vi "Test Front Panel.vi"() -> ()   [LabVIEW 2018]
uses:
  Controls/Gauge TDef.ctl
  Controls/BlockStart Button.ctl
  Controls/BlockEnd Button.ctl
  Controls/GUI_Buttons_23x22_W2K.llb/MacroPlay.ctl
  Controls/GUI_Buttons_23x22_W2K.llb/MacroPause.ctl
  Controls/GUI_Buttons_23x22_W2K.llb/MacroStop.ctl
  Controls/GUI_Buttons_23x22_W2K.llb/Delete1.ctl
  Controls/GUI_Buttons_23x22_W2K.llb/EditGroup_1.ctl
  Controls/GUI_Buttons_23x22_W2K.llb/Cut.ctl
  Controls/GUI_Buttons_23x22_W2K.llb/Copy.ctl
  Controls/GUI_Buttons_23x22_W2K.llb/Paste.ctl
  Controls/GUI_Buttons_23x22_W2K.llb/FileGroup_1.ctl
  Controls/GUI_Buttons_23x22_W2K.llb/New.ctl
  Controls/GUI_Buttons_23x22_W2K.llb/Open.ctl
  Controls/GUI_Buttons_23x22_W2K.llb/Save.ctl
  Controls/Timing Mode.ctl
  Enable Controls API.llb/Action.ctl
  Enable Controls.lvlib
panel:
  out "PID Control Within Tolerance":bool
  out "Flow Meter":bool
  out "Thermocouple":bool
  out "Agilent":bool
  out "DAQ":bool
  in  "Rest All IO":bool
  in  "Exit":bool
  in  "Tab Control":T1(tab)
  in  "Go to Next Step":bool
  in  "BP Regulator Manual Control":bool
  in  "Current Manual Control":bool caption="Current Enabled"
  in  "Open Config":bool
  in  "Delete Config":bool
  in  "New Config":bool
  in  "Current Configration File":u16(ring) items=["Default"]
  out "Actual  Voltage":dbl(slide) scale=0.0..20.0 scale format="%#_g V"
  out "Current File Name":string
  out "Actual Current":dbl(slide) scale=0.0..360.0 scale format="%#_g mA"
  in  "Control Devices":cluster{"Current":dbl, "BP Regulator":dbl} {"BP Regulator" scale=0.0..300.0 scale format="%#3_0f psig"; "Current" scale=0.0..300.0 scale format="%#_g mA"}
  out "Test Status":T2(ring)
  out "Analog Sensors":T3 {"Fuel Temp" scale=0.0..150.0 scale format="%#.1f"; "Flow(lbs/hr)" scale=0.0..1000.0 scale format="%#.1f"; "BP Monitor" scale=0.0..10.0 scale format="%#.1f"; "Bypass Pressure (psig)" scale=0.0..50.0 scale format="%#.1f"; "(Not Used)" scale=0.0..200.0 scale format="%#.1f"; "Back Pressure" scale=0.0..300.0 scale format="%#.1f"; "Diff. Pressure  (60 psid)" scale=0.0..60.0 scale format="%#.1f"; "Supply Pressure" scale=0.0..400.0 scale format="%#.1f"}
  in  "BlkMrkGrp":cluster{"Block Start":T4, "Block End":T5}
  in  "MacroGroup":T9
  in  "Delete":T10
  in  "EditGroup_1":T11
  in  "FileGroup_1":T15
  in  "Test Table":string[][](table)=[["", "20", "10", "109 ", "200", " ", " ", " ", " ", " ", " ", " ", " ", " ", " "], ["", "40", "22", "160", "200", "", " ", " ", " ", " ", " ", " ", " ", " ", " "], ["", "10", "32", "400", "500", "", " ", " ", " ", " ", " ", " ", " ", " ", " "]] caption="Current         Dwell            Min Flow       Max Flow        Actual Flow    Hysteresis"
  out "EditLine":i32=65534
  out "EditCol":i32=65534
  in  "StartTest":bool
  in  "StopTest":bool
  in  "PauseTest":bool
  out "CountDown Pie":picture
  out "CountDown Text":string="0:00"
  in  "Test Timing Mode":T19
  in  "Send to Excel":bool
  in  "Additional Report Values":cluster{"Excel  Name":string, "Value":string}[](array[cluster])
  out "Test Table2":string[][](table)=[["", "20", "10", "109 ", "200", " ", " ", " ", " ", " ", " ", " ", " ", " ", " "], ["", "40", "22", "160", "200", "", " ", " ", " ", " ", " ", " ", " ", " ", " "], ["", "10", "32", "400", "500", "", " ", " ", " ", " ", " ", " ", " ", " ", " "]] caption="Table"
  in  "template (empty)":path
  out "Parameter Table Out":string[][](table)
  out "Flow-Current XY Graph":cluster{cluster{"X":dbl, "Y":dbl}[]}[](graph)
  in  "Save Password":bool
  in  "Editor Password":string
  in  "Tolerance (psid)":dbl=50.0
  in  "PID Auto Tune":bool
  in  "reset":bool
  in  "Send PID":bool
  in  "H20 Specific Gravity (h)":dbl
  out "Current Flow Conversion Formula":string
  in  "Flow Conversion Formula":string
  out "Current  SG Calibration Formula":string
  in  "Specific Gravity Calibration Formula":string
  out "Current Calibration Formula":string
  in  "Apply Flow Formula":bool
  in  "Flow Calibration Formula":string
  in  "System Refresh Button":bool
  in  "Enable":bool
  in  "Temp Channel":refnum<k21>="Fuel_Temp"
  in  "BP Regulator Command":refnum<k21>="BP_Regulator_Command"
  in  "DAQ Sensor Channels":T20={"Supply Pressure"="Supply_Pressure", "DIff Pressure (50 psid)"="Diff_Pressure_1", "Bypass pressure"="Bypass_Pressure_3883255", "Diff Pressure (100 psid)"="Diff_Pressure_2_38883255", "BP Monitor"="Unused"}
  in  "PID_Gains.proportional gain (Kc)":dbl
  in  "PID_Gains.integral time (Ti, min)":dbl
  in  "PID_Gains.derivative time (Td, min)":dbl
  in  "Back Pressure Reg Output (Range , psid)":cluster{"OUTHI":dbl, "OUTLO":dbl}={"OUTHI"=300.0, "OUTLO"=0.0}
  in  "Setpoint (psid)":dbl=50.0
  in  "Agilent Resource Name":refnum<visa-resource-name>="Agilent"
  in  "FEM-03 Port":refnum<visa-resource-name>="COM1"
  in  "Simulate Hardware":bool=TRUE
  out "USB 6211":errorcluster
  out "USB Agilent":errorcluster
  out "USB TC 01":errorcluster
  out "FEM-03":errorcluster
  out "Parameter Table Out 2":string[][](table) caption="Parameter Table + Comment Out"
  in  "Alarms":T21={"Flow"=0.0, "Flow 2"=0.0, "Fuel Temp"=350.0, "Fuel Temp 2"=0.0, "Supply Pressure"=250.0, "Supply Pressure "=200.0, "Diff. Pressure (50psid)"=100.0, "Diff. Pressure (50psid) 2"=20.0, "Back Pressure"=100.0, "Back Pressure 2"=20.0, "Bypass Pressure"=100.0, "Bypass Pressure 2"=20.0, "Diff. Pressure (100psid)"=100.0, "Diff. Pressure (100psid) 2"=20.0, "BP (Monitor)"=0.0, "BP (Monitor) 2"=0.0}
  out "error out":errorcluster
  # "[n + offset]"
  # "-----Test Parameter Rows-------\n0-Step ID\n1-Current\n2-Dwell\n3-Min Flow\n4-Max Flow\n5-Hysteresis\n\n----TestData Rows---------\n6-Flow Rate\n7-Actual mA\n8-Temperature\nDAQ Sensor 1\nDAQ Sensor 2\nDAQ Sensor 3\n.\n.\nDAQ Sensor N"
  # "Part No."
  # "Sensor Alarms"
  # "Calibration Formulas"
  # "Y (calibrated flow) ="
  # "Y=uncal Flow (gpm)"
  # "Default= 0.2259*x**6 - 0.7962*x**5 + 1.0609*x**4 - 0.6469*x**3 + 0.2101*x**2 - 0.0444*x + 0.0004"
  # "s= Initial Specifc Gravity\nx=Initial Temp\nt=Current Temp"
  # "SG (Specific Gravity) ="
  # "Default=s +(x-t)*.0005"
  # "FLow (lb/hr)="
  # "h= H20 Specific Gravity\ns=specific gravity\nY=calibrated Flow"
  # "Default=Y*h*60*s"
  # "External Instruments"
  # "Control Parameters"
  # "DAQ Channels"
  # "Advanced Settings"
  # "LO Alarm"
  # "HI Alarm"
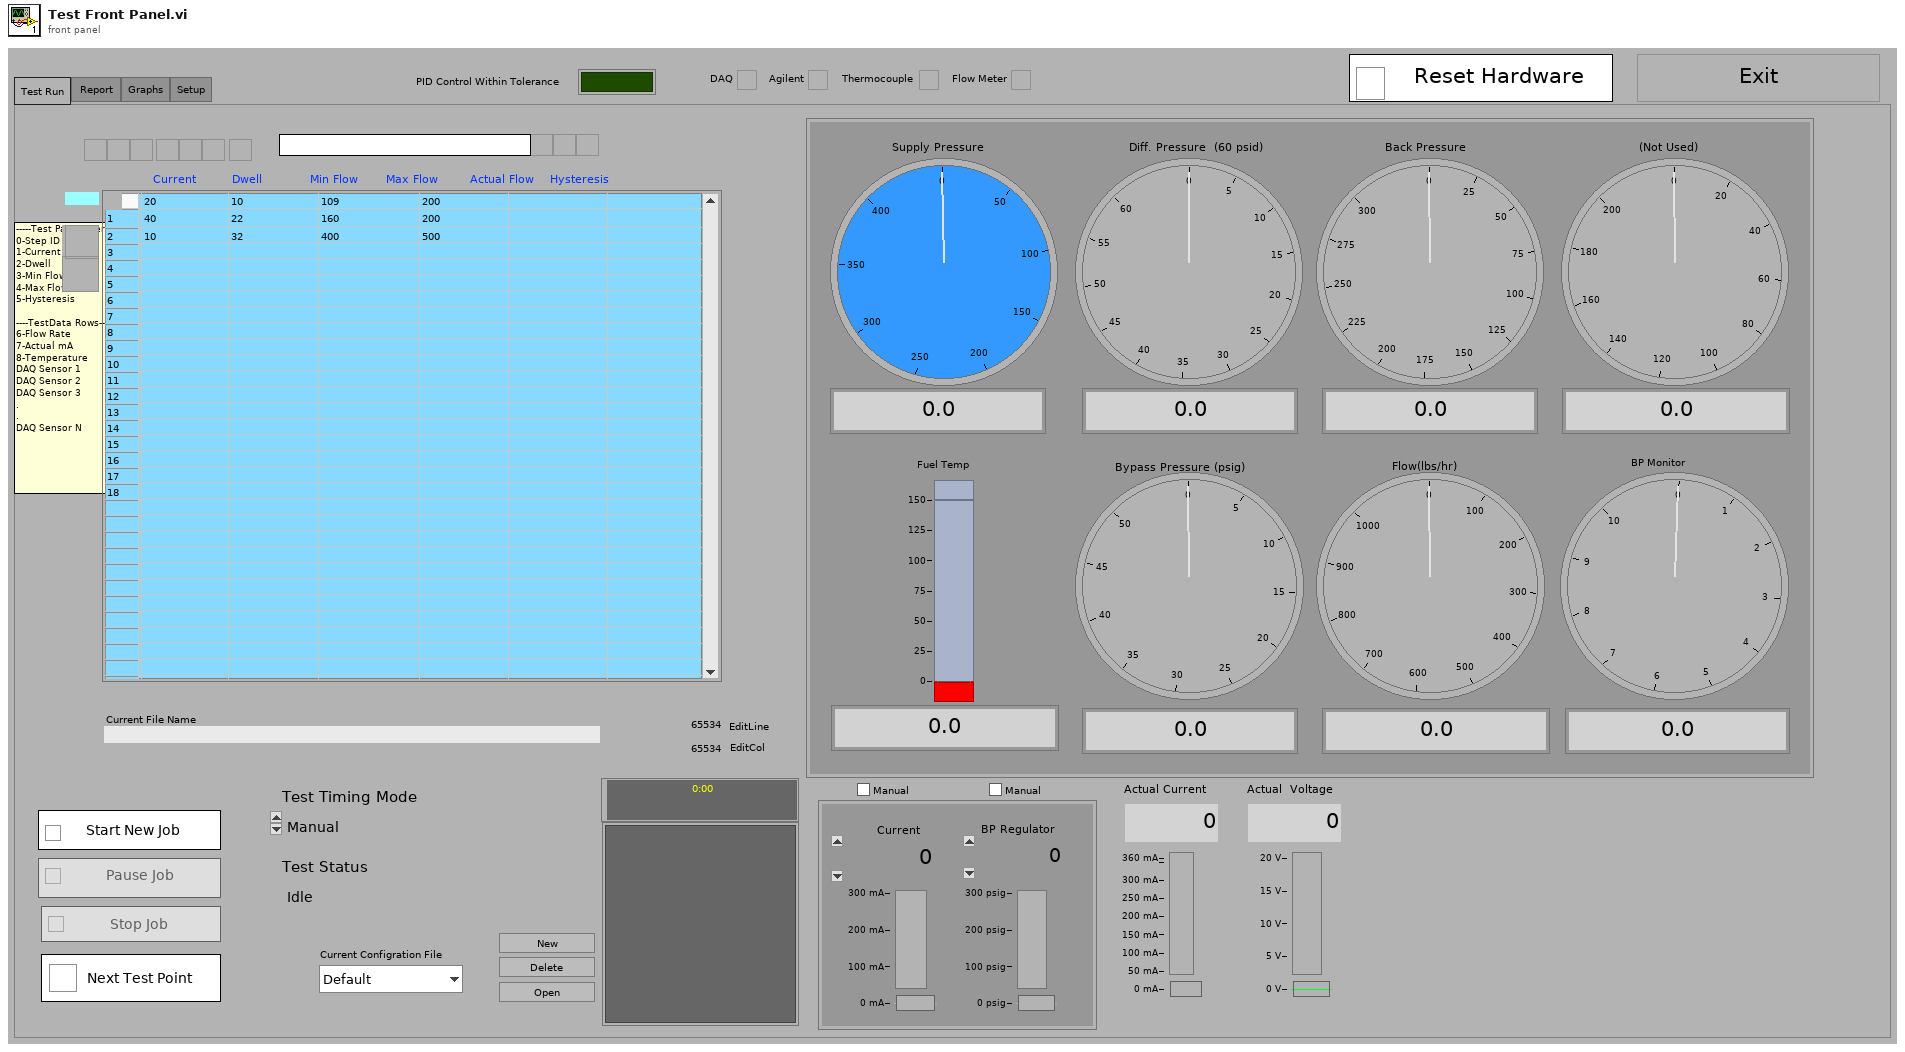
[diagram p1: front panel]
types:
  T1 = enum32{"Test Run", "Report ", "Graphs", "Setup", "Data Files"}
  T2 = enum16{"Idle", "Test Running", "Test Paused", "Test Completed"}
  T3 = typedef "Gauge TDef.ctl" = cluster{"Flow(lbs/hr)":dbl, "Fuel Temp":dbl, "Supply Pressure":dbl, "Diff. Pressure  (60 psid)":dbl, "Back Pressure":dbl, "(Not Used)":dbl, "Bypass Pressure (psig)":dbl, "BP Monitor":dbl}
  T4 = typedef "BlockStart Button.ctl" = bool
  T5 = typedef "BlockEnd Button.ctl" = bool
  T6 = typedef "MacroPlay.ctl" = bool
  T7 = typedef "MacroPause.ctl" = bool
  T8 = typedef "MacroStop.ctl" = bool
  T9 = cluster{"MacroPlay":T6, "MacroPause":T7, "MacroStop":T8, "MacroName":u16}
  T10 = typedef "Delete1.ctl" = bool
  T11 = typedef "EditGroup_1.ctl" = cluster{"Cut":T12, "Copy":T13, "Paste":T14}
  T12 = typedef "Cut.ctl" = bool
  T13 = typedef "Copy.ctl" = bool
  T14 = typedef "Paste.ctl" = bool
  T15 = typedef "FileGroup_1.ctl" = cluster{"New":T16, "Open":T17, "Save":T18}
  T16 = typedef "New.ctl" = bool
  T17 = typedef "Open.ctl" = bool
  T18 = typedef "Save.ctl" = bool
  T19 = typedef "Timing Mode.ctl" = enum16{"Manual", "Automatic", "Semi-Automatic"}
  T20 = cluster{"Supply Pressure":refnum<k21>, "DIff Pressure (50 psid)":refnum<k21>, "Bypass pressure":refnum<k21>, "Diff Pressure (100 psid)":refnum<k21>, "BP Monitor":refnum<k21>}
  T21 = cluster{"Flow":dbl, "Flow 2":dbl, "Fuel Temp":dbl, "Fuel Temp 2":dbl, "Supply Pressure":dbl, "Supply Pressure ":dbl, "Diff. Pressure (50psid)":dbl, "Diff. Pressure (50psid) 2":dbl, "Back Pressure":dbl, "Back Pressure 2":dbl, "Bypass Pressure":dbl, "Bypass Pressure 2":dbl, "Diff. Pressure (100psid)":dbl, "Diff. Pressure (100psid) 2":dbl, "BP (Monitor)":dbl, "BP (Monitor) 2":dbl}
  T22 = typedef "Enable Controls.lvlib/Action.ctl" = enum16{"Editor Init", "Init", "Operator Init", "Timed Test Start", "Manual Test Start", "Stop Test", "Close", "Set States"}
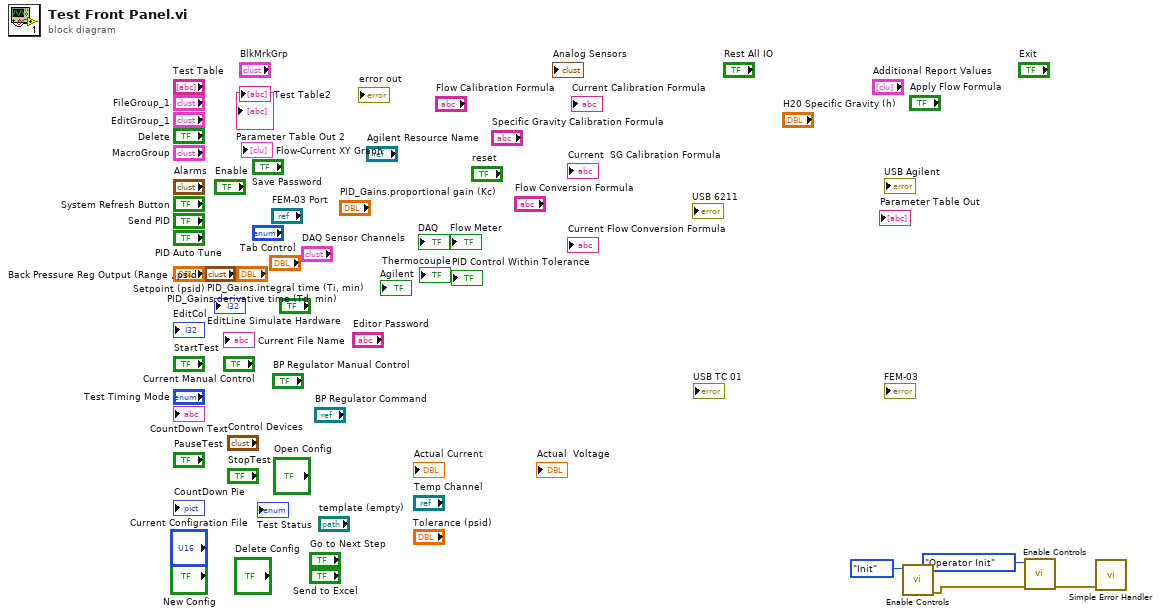
[diagram p0: block diagram]
diagram:
  n1 = call "Enable Controls.vi"("Enabled State"=Action."Init") -> ("error out"=w1:errorcluster)  [unwired: 10 in]
  n2 = call "Enable Controls.vi"("error in"=w1, "Enabled State"=Action."Operator Init") -> ("error out"=w3:errorcluster)  [unwired: 9 in]
  n3 = call <vilib>:"Simple Error Handler.vi"("error in (no error)"=w3) -> ()  [unwired: 4 in, 5 out]
